vi "Compare Old and New LSM.vi"(4 "New LSM Settings":T2={"Channel Selection"=enum."A", "Pixel Count"={"Pixels in X"=512, "Pixels in Y"=512}, "Field Size"=90.0, "Frames"=2, "Averaging"=FALSE, "Alignment"=0.0, "Scan Mode"=TRUE, "Gain"={"Gain A"=1, "Gain B"=1}, "Enable PMTs"={"A"=TRUE, "B"=TRUE}, "Voltage Range"={"Range A"=10, "Range B"=10}, "Multi Frame Count"=0.0, "Trigger Mode"=2.0, "Real Time Averaging"=TRUE, "PFOV"=0.0, "MicronsPerPx"=0.0} {"Field Size" min=5.0 max=255.0 step=1.0 scale=5.0..255.0; "PFOV" min=1.0 max=300.0 step=0.1; "MicronsPerPx" min=0.01 step=0.01 format="%.2f"; "Gain"."Gain B" min=1 max=100 step=1; "Gain"."Gain A" min=1 max=100 step=1; "Voltage Range"."Range B" items=["100mV"=5, "200mV"=6, "400mV"=7, "1V"=10, "2V"=11, "4V"=12]; "Voltage Range"."Range A" items=["100mV"=5, "200mV"=6, "400mV"=7, "1V"=10, "2V"=11, "4V"=12]; "Pixel Count"."Pixels in Y" items=["32"=32, "64"=64, "128"=128, "256"=256, "512"=512, "1024"=1024, "2048"=2048]; "Pixel Count"."Pixels in X" items=["32"=32, "64"=64, "128"=128, "256"=256, "512"=512, "1024"=1024, "2048"=2048]}, 5 "Old LSM Settings":T2={"Channel Selection"=enum."A", "Pixel Count"={"Pixels in X"=512, "Pixels in Y"=512}, "Field Size"=90.0, "Frames"=2, "Averaging"=FALSE, "Alignment"=0.0, "Scan Mode"=TRUE, "Gain"={"Gain A"=1, "Gain B"=1}, "Enable PMTs"={"A"=TRUE, "B"=TRUE}, "Voltage Range"={"Range A"=10, "Range B"=10}, "Multi Frame Count"=0.0, "Trigger Mode"=2.0, "Real Time Averaging"=TRUE, "PFOV"=0.0, "MicronsPerPx"=0.0} {"Field Size" min=5.0 max=255.0 step=1.0 scale=5.0..255.0; "PFOV" min=1.0 max=300.0 step=0.1; "MicronsPerPx" min=0.01 step=0.01 format="%.2f"; "Gain"."Gain B" min=1 max=100 step=1; "Gain"."Gain A" min=1 max=100 step=1; "Voltage Range"."Range B" items=["100mV"=5, "200mV"=6, "400mV"=7, "1V"=10, "2V"=11, "4V"=12]; "Voltage Range"."Range A" items=["100mV"=5, "200mV"=6, "400mV"=7, "1V"=10, "2V"=11, "4V"=12]; "Pixel Count"."Pixels in Y" items=["32"=32, "64"=64, "128"=128, "256"=256, "512"=512, "1024"=1024, "2048"=2048]; "Pixel Count"."Pixels in X" items=["32"=32, "64"=64, "128"=128, "256"=256, "512"=512, "1024"=1024, "2048"=2048]}) -> (0 "LSM Settings with index of change":T3 {"New LSM Settings"."Field Size" min=5.0 max=255.0 step=1.0 scale=5.0..255.0; "New LSM Settings"."PFOV" min=1.0 max=300.0 step=0.1; "New LSM Settings"."MicronsPerPx" min=0.01 step=0.01 format="%.2f"; "New LSM Settings"."Gain"."Gain B" min=1 max=100 step=1; "New LSM Settings"."Gain"."Gain A" min=1 max=100 step=1; "New LSM Settings"."Voltage Range"."Range B" items=["100mV"=5, "200mV"=6, "400mV"=7, "1V"=10, "2V"=11, "4V"=12]; "New LSM Settings"."Voltage Range"."Range A" items=["100mV"=5, "200mV"=6, "400mV"=7, "1V"=10, "2V"=11, "4V"=12]; "New LSM Settings"."Pixel Count"."Pixels in Y" items=["32"=32, "64"=64, "128"=128, "256"=256, "512"=512, "1024"=1024, "2048"=2048]; "New LSM Settings"."Pixel Count"."Pixels in X" items=["32"=32, "64"=64, "128"=128, "256"=256, "512"=512, "1024"=1024, "2048"=2048]})   [LabVIEW 2020]
uses:
  _Controls/Confocal Controls.ctl
  _Globals/Global Controls.vi
panel:
  out "LSM CF":T1
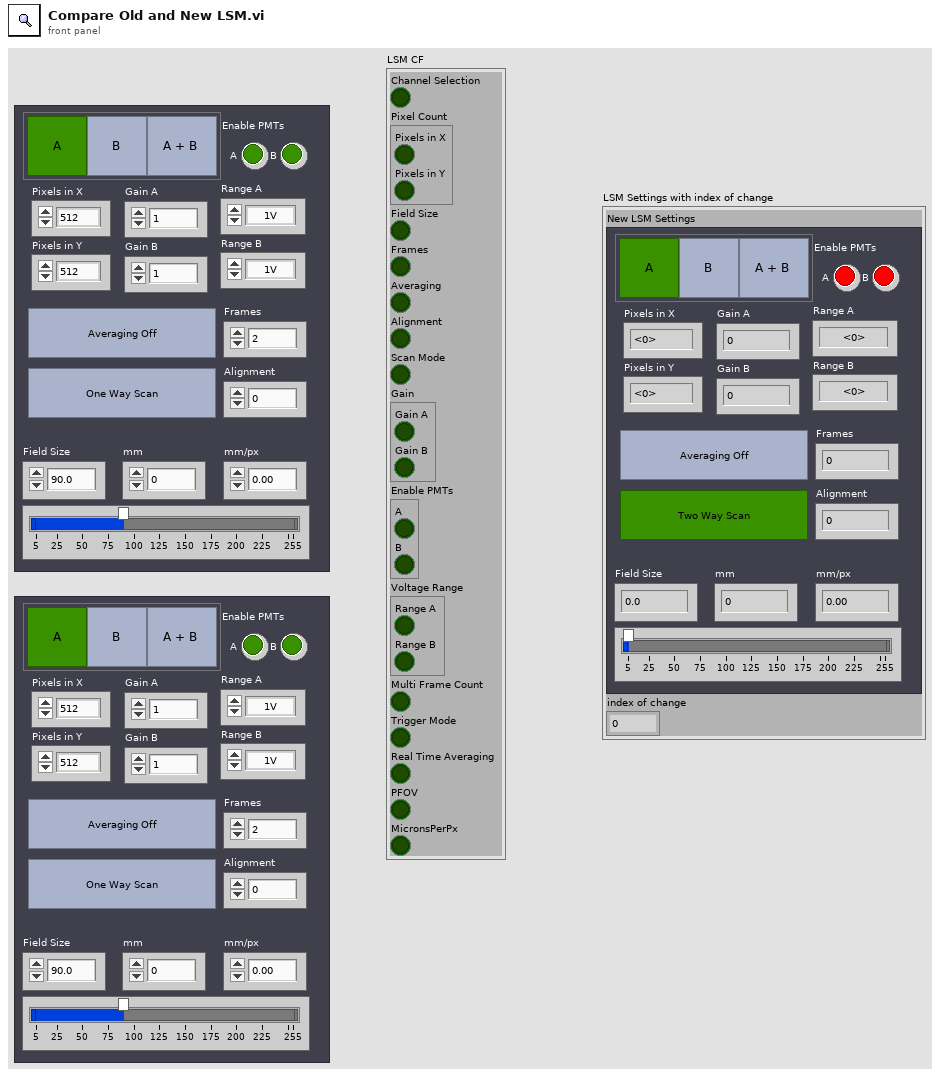
[diagram p1: front panel]
types:
  T1 = cluster{"Channel Selection":bool, "Pixel Count":cluster{"Pixels in X":bool, "Pixels in Y":bool}, "Field Size":bool, "Frames":bool, "Averaging":bool, "Alignment":bool, "Scan Mode":bool, "Gain":cluster{"Gain A":bool, "Gain B":bool}, "Enable PMTs":cluster{"A":bool, "B":bool}, "Voltage Range":cluster{"Range A":bool, "Range B":bool}, "Multi Frame Count":bool, "Trigger Mode":bool, "Real Time Averaging":bool, "PFOV":bool, "MicronsPerPx":bool}
  T2 = typedef "Confocal Controls.ctl" = cluster{"Channel Selection":enum32{"A", "B", "AB"}, "Pixel Count":cluster{"Pixels in X":u32, "Pixels in Y":u32}, "Field Size":dbl, "Frames":u8, "Averaging":bool, "Alignment":dbl, "Scan Mode":bool, "Gain":cluster{"Gain A":u8, "Gain B":u8}, "Enable PMTs":cluster{"A":bool, "B":bool}, "Voltage Range":cluster{"Range A":u16, "Range B":u16}, "Multi Frame Count":dbl, "Trigger Mode":dbl, "Real Time Averaging":bool, "PFOV":dbl, "MicronsPerPx":dbl}
  T3 = cluster{"New LSM Settings":T2, "index of change":i32}
  T4 = typedef "Tweezertron Ctrl Refs.ctl" = cluster{"LSM Settings":refnum<vi>, "iFlex Control":refnum<vi>, "PIFOC Settings":refnum<vi>, "PinSelector":refnum<vi>, "Manlight Controls":refnum<vi>, "Exp Params":refnum<vi>, "Image Thresholds":refnum<vi>, "RevFrame":refnum<vi>, "Spots":refnum<vi>}
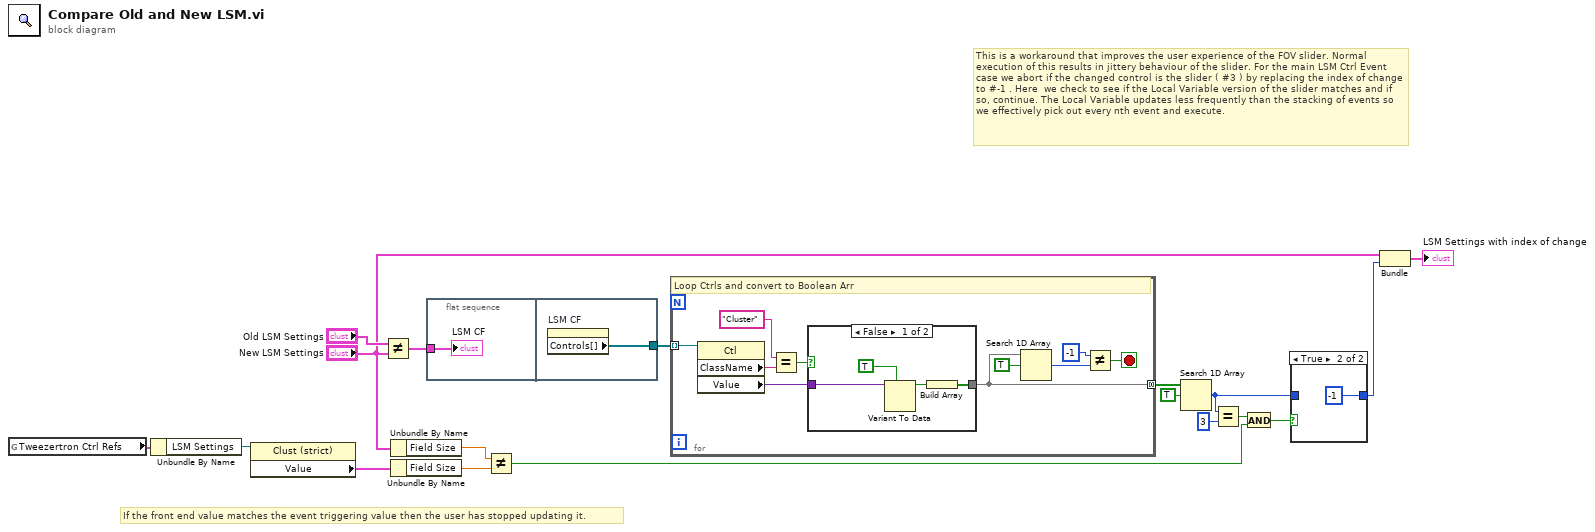
[diagram p0: block diagram]
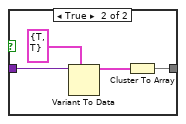
[diagram p3: hidden frame]
diagram:
  # "If the front end value matches the event triggering value then the user has stopped updating it."
  # "This is a workaround that improves the user experience of the FOV slider. Normal execution of this results in jittery behaviour of the slider. For the main LSM Ctrl Event case we abort if the changed control is the slider ( #3 ) by replacing the index of change to #-1 . Here  we check to see if the Local Variable version of the slider matches and if so, continue. The Local Variable updates less frequently than the stacking of events so we effectively pick out every nth event and execute."
  n1 = global read "Global Controls.vi" "Tweezertron Ctrl Refs"() -> (w4:T4)
  n2 = Unbundle By Name(w4) -> ("LSM Settings"=w3:refnum<vi>)
  n3 = property class="Clust (strict)"(reference=w3) -> ("Value"=w2:T2)  [unwired: 1 in, 2 out]
  n4 = Not Equal?(x="Old LSM Settings", y="New LSM Settings") -> (x != y?=w10:T1)
  n5 = Unbundle By Name("New LSM Settings") -> ("Field Size"=w8:dbl)
  n6 = Unbundle By Name(w2) -> ("Field Size"=w1:dbl)
  n7 = flat-sequence {
    tunnel: w10 -> [w19]
    tunnel: [w20] -> w15
    frame #0 {
      "LSM CF" <- w19
    }
    frame #1 {
      n8 = property on="LSM CF" class="Clust (strict)"() -> ("Controls[]"=w20:refnum<vi>[])  [unwired: 2 in, 2 out]
    }
  }
  n9 = Not Equal?(x=w8, y=w1) -> (x != y?=w5:bool)
  n10 = for {
    tunnel: w15 -> [w30] mode=indexing
    tunnel: [w24] -> w17 mode=concatenating
    stop <- w21 stop-if-true
    # "Loop Ctrls and convert to Boolean Arr"
    n11 = property class="Ctl"(reference=w30) -> ("ClassName"=w27:string, "Value"=w26:variant)  [unwired: 1 in, 2 out]
    n12 = Equal?(x="Cluster", y=w27) -> (x = y?=w29:bool)
    n13 = case shown="False" w29 {
      tunnel: w26 -> [w34 w38]
      tunnel: [w31 w35] -> w24
      frame False {
        n14 = Variant To Data(type=TRUE, Variant=w34) -> (data=w32:bool)  [unwired: 1 in, 1 out]
        n15 = Build Array(w32) -> (w31:bool[])
      }
      frame True {
        n16 = Variant To Data(type=cluster{bool, bool} {TRUE, TRUE}, Variant=w38) -> (data=w36:cluster{bool, bool})  [unwired: 1 in, 1 out]
        n17 = Cluster To Array(cluster=w36) -> (array=w35:bool[])
      }
    }
    n18 = Search 1D Array(1D array=w24, element=TRUE) -> (index of element=w23:i32)  [unwired: 1 in]
    n19 = Not Equal?(x=-1, y=w23) -> (x != y?=w21:bool)
  }
  n20 = Search 1D Array(1D array=w17, element=TRUE) -> (index of element=w12:i32)  [unwired: 1 in]
  n21 = Equal?(x=w12, y=3) -> (x = y?=w7:bool)
  n22 = And(x=w7, y=w5) -> (x .and. y?=w6:bool)
  n23 = case shown="True" w6 {
    tunnel: [w39 -1 ("x")] -> w13
    tunnel: w12 -> [w39 _]
    frame False {
    }
    frame True {
    }
  }
  n24 = Bundle("New LSM Settings"="New LSM Settings", "x"=w13) -> (→"LSM Settings with index of change":cluster{"New LSM Settings":T2, "x":i32})  [unwired: 1 in]
